vi "SeqMgr.Variables, Populate Array Indices.vi"(8 "error in":errorcluster, 10 "String":string, 11 "Variables":variant) -> (0 "error out":errorcluster, 2 "String Out":string, 3 "Variables Out":variant)   [LabVIEW 2024, in "EQMF.lvlib" / "SeqMgr.lvlib"]
uses:
  SeqMgr.lvlib
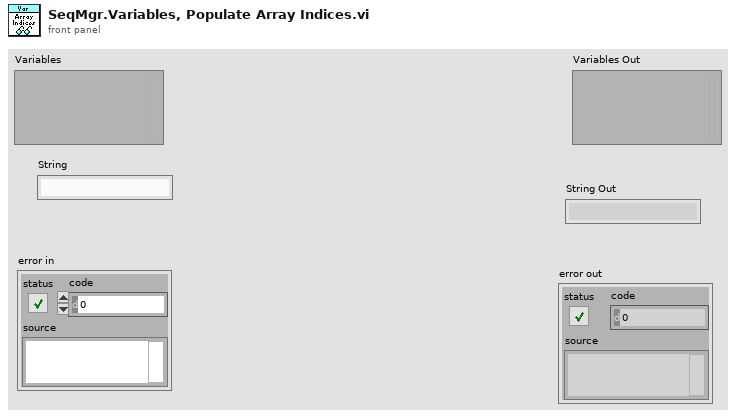
[diagram p1: front panel]
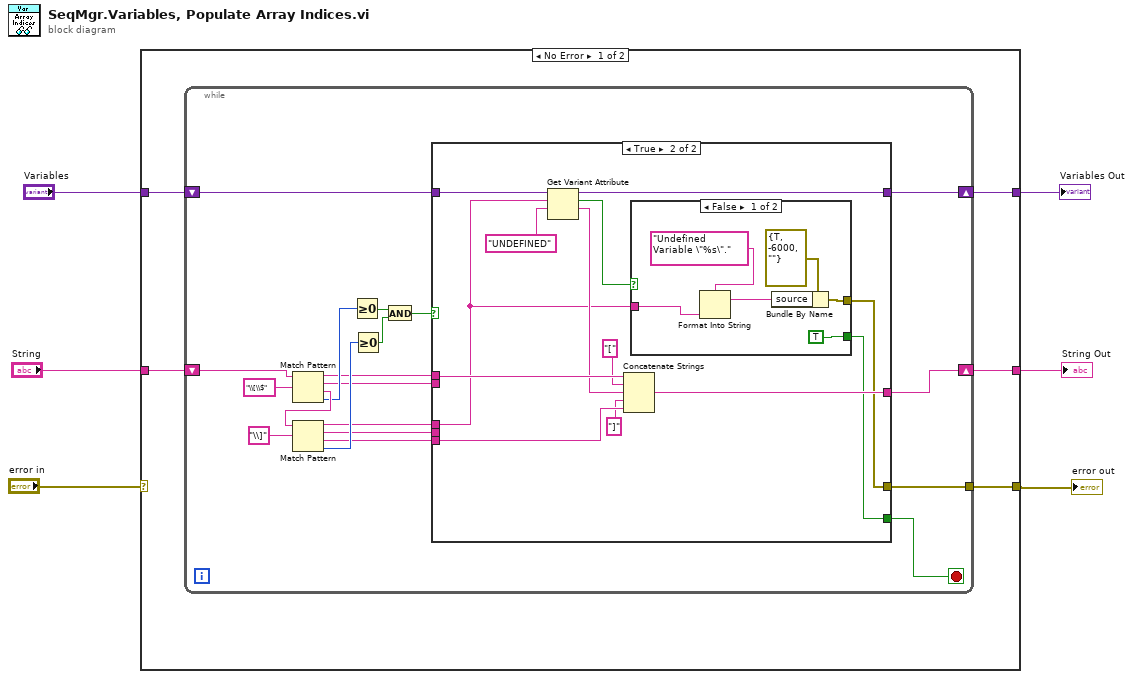
[diagram p0: block diagram]
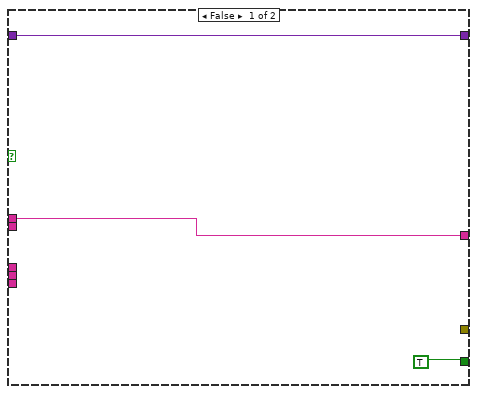
[diagram p2: hidden frame]
diagram:
  n1 = case shown="No Error" "error in" {
    selector: "error in" -> [_ w53]
    tunnel: "Variables" -> [w11 w55]
    tunnel: [w10 w55] -> w6
    tunnel: "String" -> [w9 w54]
    tunnel: [w8 w54] -> w4
    tunnel: [w7 w53] -> w2
    frame No Error {
      n2 = while {
        shift-right: [w29] -> w10
        shift-left: w11 -> [w30]
        shift-right: [w14] -> w8
        shift-left: w9 -> [w21]
        tunnel: [w12] -> w7
        stop <- w13 stop-if-true
        n3 = Match Pattern(string=w21, regular expression="\\[\\$") -> (before substring=w19:string, match substring=w18:string, after substring=w26:string, offset past match=w25:i32)  [unwired: 1 in]
        n4 = Match Pattern(string=w26, regular expression="\\]") -> (before substring=w20:string, match substring=w17:string, after substring=w16:string, offset past match=w24:i32)  [unwired: 1 in]
        n5 = Greater Or Equal To 0?(x=w25) -> (x >= 0?=w23:bool)
        n6 = Greater Or Equal To 0?(x=w24) -> (x >= 0?=w22:bool)
        n7 = And(x=w23, y=w22) -> (x .and. y?=w15:bool)
        n8 = case shown="True" w15 {
          tunnel: w30 -> [w31 w46]
          tunnel: [w31 w45] -> w29
          tunnel: w20 -> [_ w34]
          tunnel: w19 -> [w32 w43]
          tunnel: w18 -> [_ _]
          tunnel: w17 -> [_ _]
          tunnel: w16 -> [_ w41]
          tunnel: [w32 w38] -> w14
          tunnel: [TRUE w36] -> w13
          tunnel: [_ w35] -> w12
          frame False {
          }
          frame True {
            n9 = Get Variant Attribute(Variant=w46, name=w34, default value (empty Variant)="UNDEFINED") -> (duplicate Variant=w45:variant, found=w37:bool, value=w42:string)  [unwired: 1 in, 1 out]
            n10 = Concatenate Strings(w43, "[", w42, "]", w41) -> (w38:string)
            n11 = case shown="False" w37 {
              tunnel: [TRUE _] -> w36
              tunnel: [w50 _] -> w35
              tunnel: w34 -> [w48 _]
              frame False {
                n12 = Format Into String(format string="Undefined Variable \"%s\"." ("source"), w48) -> (resulting string=w47:string)  [unwired: 2 in, 1 out]
                n13 = Bundle By Name(cluster=errorcluster {"status"=TRUE, "code"=-6000, "source"=""} ("error constant"), "source"=w47) -> (w50:errorcluster)
              }
              frame True {
              }
            }
          }
        }
      }
    }
    frame Error {
    }
  }
  "Variables Out" <- w6
  "String Out" <- w4
  "error out" <- w2
